vi "viSendSerialData.vi"(2 "error in (no error)":errorcluster, 3 "input variable":u8[](array[numeric]), 4 "VISA resource name in":refnum<visa-resource-name>) -> (0 "error out":errorcluster, 1 "VISA resource name out":refnum<visa-resource-name>)   [LabVIEW 2009]
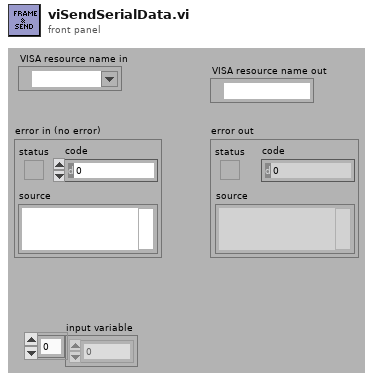
[diagram p1: front panel]
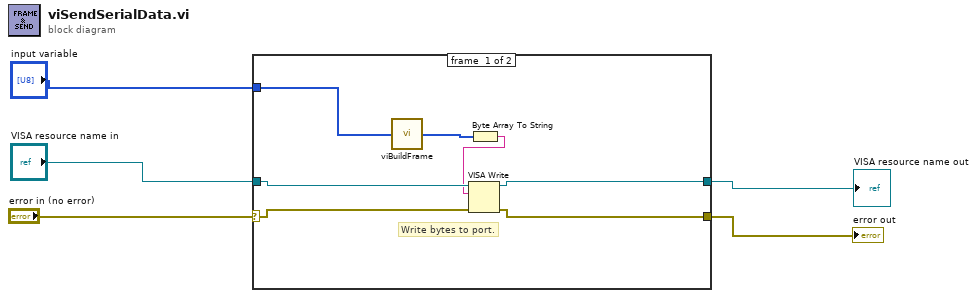
[diagram p0: block diagram]
diagram:
  n1 = case "Read bytes from port." shown="No Error" "error in (no error)" {
    selector: "error in (no error)" -> [w11 w13]
    tunnel: [w9 w13] -> w2
    tunnel: [w10 w14] -> w5
    tunnel: "VISA resource name in" -> [w12 w14]
    tunnel: "input variable" -> [w8 _]
    frame #0 {
      # "Write bytes to port."
      n2 = call "viBuildFrame.vi"("input variable"=w8) -> ("output bytes"=w7:u8[])
      n3 = Byte Array To String(unsigned byte array=w7) -> (string=w6:string)
      n4 = VISA Write(VISA resource name=w12, write buffer=w6, error in (no error)=w11) -> (VISA resource name out=w10:refnum<visa-resource-name>, error out=w9:errorcluster)  [unwired: 1 out]
    }
    frame #1 {
      # "Error occurred \nreading Bytes at \nSerial Port"
    }
  }
  "error out" <- w2
  "VISA resource name out" <- w5
